vi "WriteBytes.vi"(8 "Uart Input":cluster{u64} {"?" format="%x"}, 10 "Data Buffer":u8[](array[numeric]), 11 "Error Input":errorcluster) -> (0 "Uart Output":cluster{u64} {"?" format="%x"}, 2 "Bytes Written":i32, 3 "Error Output":errorcluster)   [LabVIEW 2019]
doc: "<B>Write</B> the <B>Data Buffer</B> (array of U8) to the serial port."
uses:
  dll/LabViewUart.dll
panel:
  # "Write Data Buffer to serial port"
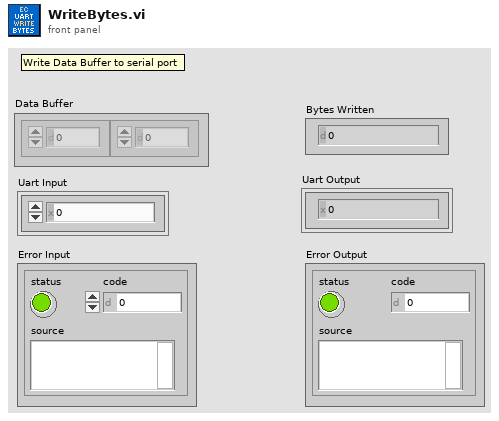
[diagram p1: front panel]
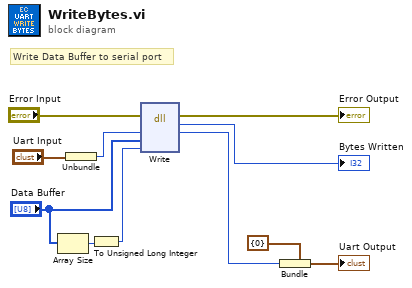
[diagram p0: block diagram]
diagram:
  # "Write Data Buffer to serial port"
  n1 = Array Size(array="Data Buffer") -> (size(s)=w7:i32)
  n2 = Unbundle("Uart Input") -> (w2:u64)
  n3 = To Unsigned Long Integer(number=w7) -> (unsigned 32bit integer=w6:u32)
  n4 = dll-call lib="D:/Google Drive/INC-2020/INC352/INC352-2020/LabVIEW/examples/uart-cmdex/SubVI/dll/LabViewUart.dll" fn="Write"(error in="Error Input", "Uart Handle"=w2, "Data Buffer"="Data Buffer", "Length"=w6) -> (error out=→"Error Output":errorcluster, "Bytes Writteb"=→"Bytes Written":i32, "Uart Handle"=w1:u64)  [unwired: 4 in, 1 out]
  n5 = Bundle(cluster=cluster{u64} {0}, w1) -> (→"Uart Output":cluster{u64})
